vi "Computer.vi"() -> ()   [LabVIEW 2015]
uses:
  <vilib>/Utility/inputDevices.llb/joystickAcquire.vi
  <vilib>/Utility/inputDevices.llb/closeJoystick.vi
panel:
  out "Robot":bool
  out "Xbox Controller":bool
  in  "Stop VI":bool
  out "TX Data":T1
  in  "ESTOP":bool
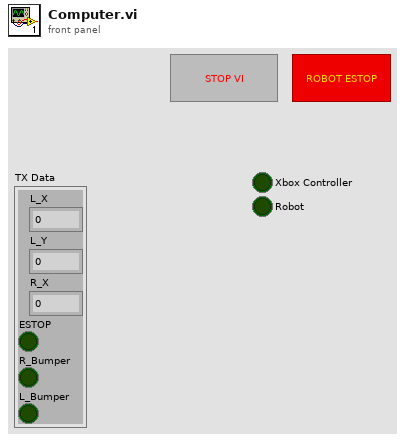
[diagram p1: front panel]
types:
  T1 = cluster{"L_X":i32, "L_Y":i32, "R_X":i32, "ESTOP":bool, "R_Bumper":bool, "L_Bumper":bool}
  T2 = cluster{"X axis":i32, "Y axis":i32, "Z axis":i32, "X axis rotation":i32, "Y axis rotation":i32, "Z axis rotation":i32, "U axis":i32, "V axis":i32}
  T3 = cluster{"button 1":bool, "button 2":bool, "button 3":bool, "button 4":bool, "button 5":bool, "button 6":bool, "button 7":bool, "button 8":bool, "button 9":bool, "button 10":bool, "button 11":bool, "button 12":bool, "button 13":bool, "button 14":bool, "button 15":bool, "button 16":bool, "button 17":bool, "button 18":bool, "button 19":bool, "button 20":bool, "button 21":bool, "button 22":bool, "button 23":bool, "button 24":bool, "button 25":bool, "button 26":bool, "button 27":bool, "button 28":bool, "button 29":bool, "button 30":bool, "button 31":bool, "button 32":bool}
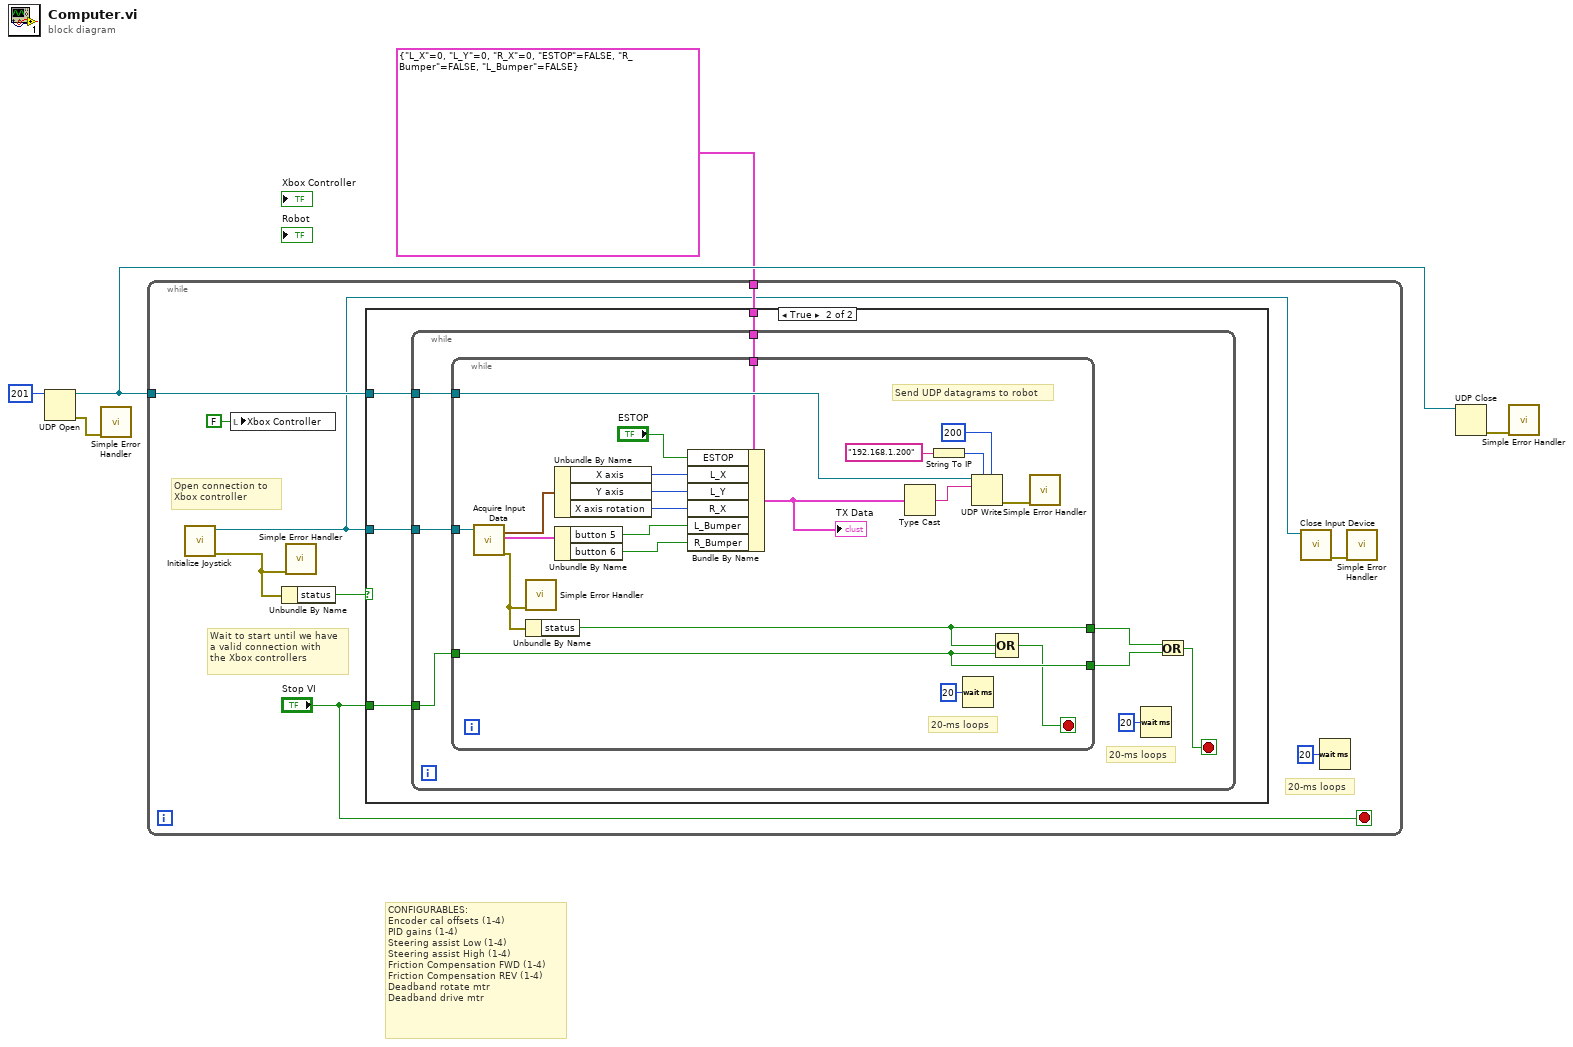
[diagram p0: block diagram]
diagram:
  # "CONFIGURABLES:\nEncoder cal offsets (1-4)\nPID gains (1-4)\nSteering assist Low (1-4)\nSteering assist High (1-4)\nFriction Compensation FWD (1-4)\nFriction Compensation REV (1-4)\nDeadband rotate mtr\nDeadband drive mtr"
  n1 = UDP Open(11:u16 201 ("port")) -> (port=w4:refnum<k16>, 0:w2:errorcluster)  [unwired: 4 in, 1 out]
  n2 = call <vilib>:"Simple Error Handler.vi"("error in (no error)"=w2) -> ()  [unwired: 4 in, 5 out]
  n3 = while {
    tunnel: w4 -> [w9]
    tunnel: T1 {"L_X"=0, "L_Y"=0, "R_X"=0, "ESTOP"=FALSE, "R_Bumper"=FALSE, "L_Bumper"=FALSE} -> [w8]
    stop <- "Stop VI" stop-if-true
    # "20-ms loops"
    # "Wait to start until we have\na valid connection with\nthe Xbox controllers"
    # "Open connection to\nXbox controller"
    n4 = call <vilib>:"Initialize Joystick.vi"() -> ("error out"=w7:errorcluster, "device ID"=w6:refnum<k1>)  [unwired: 10 in]
    n5 = local write "Xbox Controller"(FALSE ("Xbox Controller")) -> ()
    n6 = Unbundle By Name(w7) -> ("status"=w14:bool)
    n7 = call <vilib>:"Simple Error Handler.vi"("error in (no error)"=w7) -> ()  [unwired: 4 in, 5 out]
    n8 = case shown="True" w14 {
      tunnel: w6 -> [_ w18]
      tunnel: "Stop VI" -> [_ w17]
      tunnel: w9 -> [_ w16]
      tunnel: w8 -> [_ w15]
      frame False {
      }
      frame True {
        n9 = while {
          tunnel: w18 -> [w25]
          tunnel: w17 -> [w24]
          tunnel: w16 -> [w22]
          tunnel: w15 -> [w21]
          stop <- w26 stop-if-true
          # "20-ms loops"
          n10 = while {
            tunnel: w25 -> [w47]
            tunnel: w24 -> [w30]
            tunnel: w22 -> [w37]
            tunnel: w21 -> [w33]
            tunnel: [w31] -> w20
            tunnel: [w30] -> w19
            stop <- w27 stop-if-true
            # "Send UDP datagrams to robot"
            # "20-ms loops"
            n11 = call-poly <vilib>:"Acquire Input Data.vi"("device ID"=w47) -> ("axis info"=w46:T2, "button info"=w45:T3, "error out"=w28:errorcluster)  [unwired: 14 in, 2 out]
            n12 = call <vilib>:"Simple Error Handler.vi"("error in (no error)"=w28) -> ()  [unwired: 4 in, 5 out]
            n13 = Unbundle By Name(w28) -> ("status"=w31:bool)
            n14 = Unbundle By Name(w46) -> ("X axis"=w42:i32, "Y axis"=w43:i32, "X axis rotation"=w44:i32)
            n15 = Unbundle By Name(w45) -> ("button 5"=w40:bool, "button 6"=w39:bool)
            n16 = Bundle By Name(cluster=w33, "ESTOP"="ESTOP", "L_X"=w42, "L_Y"=w43, "R_X"=w44, "L_Bumper"=w40, "R_Bumper"=w39) -> (w32:T1)
            "TX Data" <- w32
            n17 = Type Cast(x=w32) -> (*(type *) &x=w38:string)  [unwired: 1 in]
            n18 = String To IP(1:"192.168.1.200" ("name")) -> (0:w36:u32)
            n19 = Wait (ms)(milliseconds to wait=u32 20) -> ()  [unwired: 1 out]
            n20 = UDP Write(address=w36, port or service name=u16 200, connection ID=w37, data in=w38) -> (error out=w29:errorcluster)  [unwired: 2 in, 1 out]
            n21 = Compound Arithmetic op=OR(w31, w30) -> (w27:bool)  [unwired: 1 in]
            n22 = call <vilib>:"Simple Error Handler.vi"("error in (no error)"=w29) -> ()  [unwired: 4 in, 5 out]
          }
          n23 = Wait (ms)(milliseconds to wait=u32 20) -> ()  [unwired: 1 out]
          n24 = Or(x=w20, y=w19) -> (x .or. y?=w26:bool)
        }
      }
    }
    n25 = call-poly <vilib>:"Close Input Device.vi"("device ID"=w6) -> ("error out"=w13:errorcluster)  [unwired: 9 in]
    n26 = Wait (ms)(milliseconds to wait=u32 20) -> ()  [unwired: 1 out]
    n27 = call <vilib>:"Simple Error Handler.vi"("error in (no error)"=w13) -> ()  [unwired: 4 in, 5 out]
  }
  n28 = UDP Close(connection ID=w4) -> (error out=w1:errorcluster)  [unwired: 1 in, 1 out]
  n29 = call <vilib>:"Simple Error Handler.vi"("error in (no error)"=w1) -> ()  [unwired: 4 in, 5 out]
